vi "Move to Origin.vi"(2 "Error In":errorcluster) -> (0 "Error Out":errorcluster)   [LabVIEW 2012]
doc: "This VI will move the front panel of the calling VI back to the orign. This should be used in the initlization of a User Interface VI."
uses:
  <vilib>/Utility/miscctls.llb/LVPointTypeDef.ctl
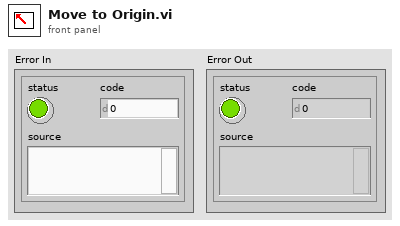
[diagram p1: front panel]
types:
  T1 = typedef "LVPointTypeDef.ctl" = cluster{"Horizontal":i16, "Vertical":i16}
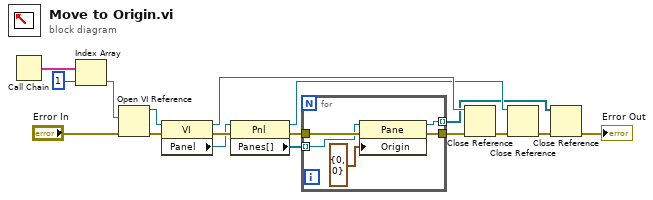
[diagram p0: block diagram]
diagram:
  n1 = Call Chain() -> (call chain=w7:string[])
  n2 = Index Array(array=w7, index=1) -> (element=w5:string)
  n3 = Open VI Reference(vi path=w5, error in (no error)="Error In") -> (vi reference=w4:refnum<vi>, error out=w3:errorcluster)  [unwired: 4 in]
  n4 = property class="VI"(reference=w4, error in=w3) -> (reference out=w13:refnum<vi>, error out=w15:errorcluster, "Panel"=w14:refnum<vi>)
  n5 = property class="Pnl"(reference=w14, error in=w15) -> (reference out=w10:refnum<vi>, error out=w17:errorcluster, "Panes[]"=w16:refnum<vi>[])
  n6 = for {
    tunnel: w16 -> [w18] mode=indexing
    tunnel: w17 -> [w22]
    tunnel: [w20] -> w12
    tunnel: [w19] -> w8 mode=indexing
    n7 = property class="Pane"(reference=w18, error in=w22, "Origin"=T1 {"Horizontal"=0, "Vertical"=0}) -> (reference out=w19:refnum<vi>, error out=w20:errorcluster)
  }
  n8 = Close Reference(reference=w13, error in (no error)=w12) -> (error out=w11:errorcluster)
  n9 = Close Reference(reference=w10, error in (no error)=w11) -> (error out=w9:errorcluster)
  n10 = Close Reference(reference=w8, error in (no error)=w9) -> (error out=→"Error Out":errorcluster)
